vi "CNTRLR - FGV Timer.vi"(7 "Timer CMD":T1, 8 "error in (no error)":errorcluster, 10 "Target Time":dbl) -> (0 "error out":errorcluster, 1 "Elapsed?":bool, 2 "Elapsed Time":dbl)   [LabVIEW 2017]
doc: "Pausable Timer based on Functional Global Variable."
uses:
  Controls/CNTRLR - Timer CMD.ctl
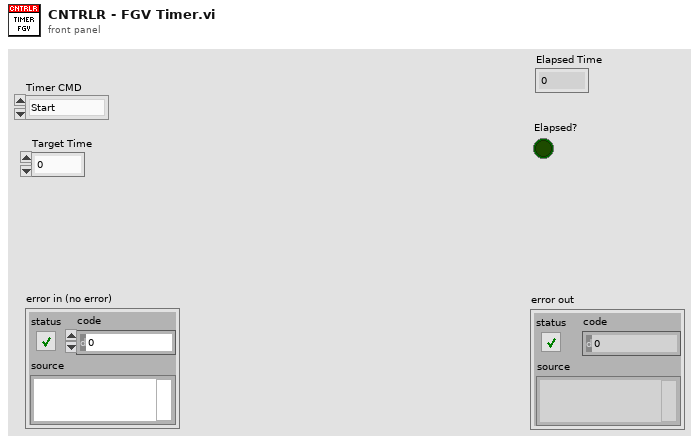
[diagram p1: front panel]
types:
  T1 = typedef "CNTRLR - Timer CMD.ctl" = enum16{"Start", "Get Time", "Pause", "Unpause"}
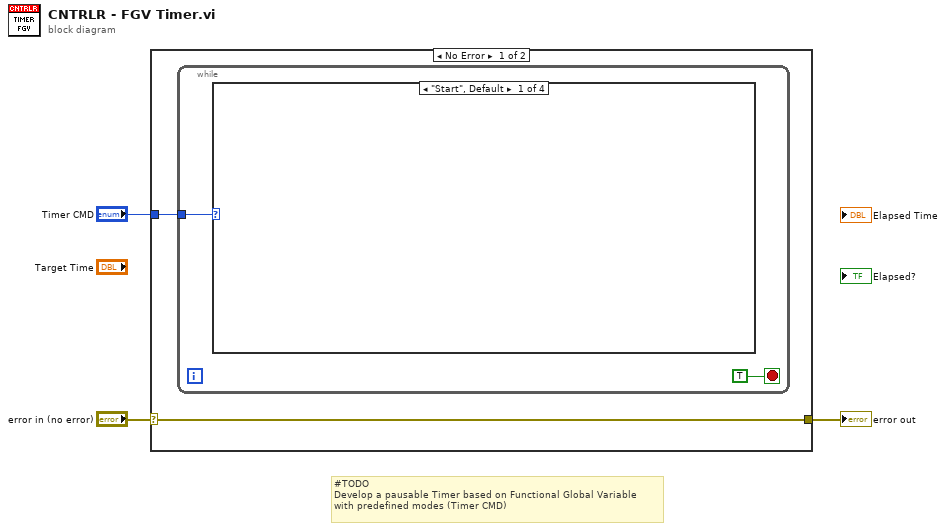
[diagram p0: block diagram]
diagram:
  # "#TODO\nDevelop a pausable Timer based on Functional Global Variable\nwith predefined modes (Timer CMD)"
  n1 = case shown="No Error" "error in (no error)" {
    selector: "error in (no error)" -> [w5 w8]
    tunnel: [w5 w8] -> w2
    tunnel: "Timer CMD" -> [w4 _]
    frame No Error {
      n2 = while {
        tunnel: w4 -> [w7]
        stop <- TRUE stop-if-true
        n3 = case shown="\"Start\", Default" w7 {
          frame "Start", Default {
          }
          frame "Get Time" {
          }
          frame "Pause" {
          }
          frame "Unpause" {
          }
        }
      }
    }
    frame Error {
    }
  }
  "error out" <- w2
